vi "Digital port disable alternative functions.vi"(8 "error in (no error)":errorcluster, 10 "Lines":T1 items=["DIO1...8"=1, "DIO9...16"=2, "DIO17...24"=3, "DIO25...32"=4], 11 "Connection ID":i32) -> (0 "error out":errorcluster, 3 "connection ID out":i32)   [LabVIEW 2009, in "MicroDAQ.lvlib" / "Digital Input.lvclass"]
uses:
  <instrlib>/MicroDAQ/Channel/Digital Input/Digital Input.lvclass
  <instrlib>/MicroDAQ/Tools/Digital IO channels.ctl
  <instrlib>/MicroDAQ/Tools/DIO Alternative functions.ctl
  <instrlib>/MicroDAQ/Tools/DIO set function argument.ctl
  <instrlib>/MicroDAQ/MicroDAQ.lvlib
  <instrlib>/MicroDAQ/Mlink library wraper/mlink.lvlib
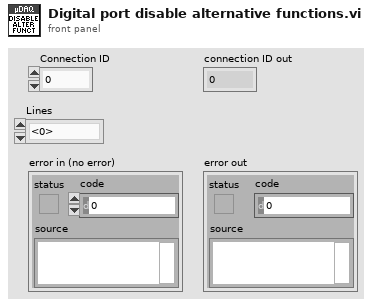
[diagram p1: front panel]
types:
  T1 = typedef "MicroDAQ.lvlib/Digital IO channels.ctl" = u8
  T2 = typedef "MicroDAQ.lvlib/DIO Alternative functions.ctl" = enum8{"None", "ENC1 (DIO1,DIO2)", "ENC2 (DIO3, DIO4)", "PWM1 (DIO10, DIO11)", "PWM2 (DIO12, DIO13)", "PWM3 (DIO14, DIO15)", "UART (DIO8-Rx, DIO9-Tx)"}
  T3 = typedef "MicroDAQ.lvlib/DIO set function argument.ctl" = enum8{"Disable", "Enable"}
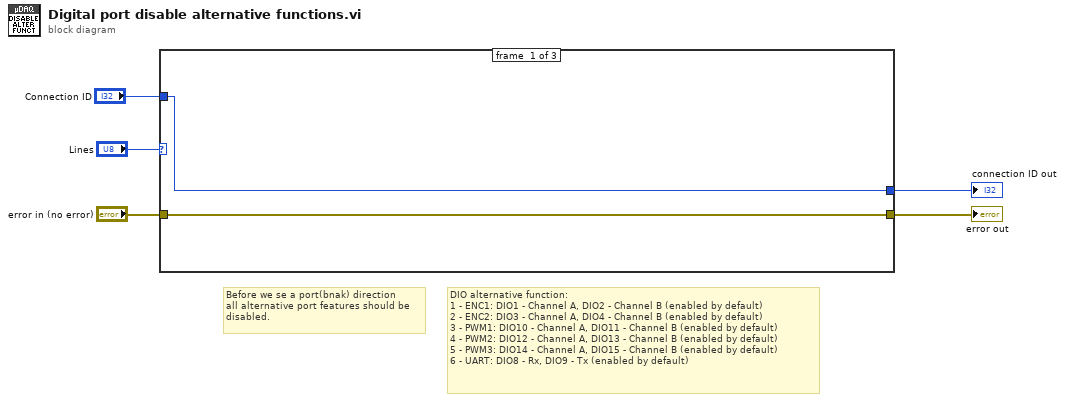
[diagram p0: block diagram]
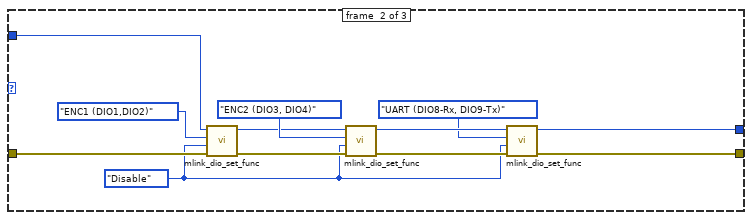
[diagram p2: hidden frame]
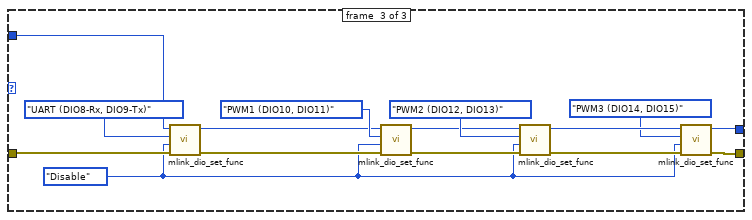
[diagram p3: hidden frame]
diagram:
  # "Before we se a port(bnak) direction\nall alternative port features should be \ndisabled."
  # "DIO alternative function:\n1 - ENC1: DIO1 - Channel A, DIO2 - Channel B (enabled by default)\n2 - ENC2: DIO3 - Channel A, DIO4 - Channel B (enabled by default)\n3 - PWM1: DIO10 - Channel A, DIO11 - Channel B (enabled by default)\n4 - PWM2: DIO12 - Channel A, DIO13 - Channel B (enabled by default)\n5 - PWM3: DIO14 - Channel A, DIO15 - Channel B (enabled by default)\n6 - UART: DIO8 - Rx, DIO9 - Tx (enabled by default)"
  n1 = case shown="2" "Lines" {
    tunnel: "Connection ID" -> [w7 w19 w23]
    tunnel: "error in (no error)" -> [w6 w18 w24]
    tunnel: [w6 w9 w26] -> w4
    tunnel: [w7 w8 w27] -> w3
    frame #0 {
    }
    frame #1 {
      w10 = DIO_set_function_argument."Disable" ("state")
      n2 = call <instrlib>:"mlink_dio_set_func.vi"("error in (no error)"=w18, "state"=w10, "function"=DIO_Alternative_functions."ENC1 (DIO1,DIO2)", "connection ID"=w19) -> ("error out"=w14:errorcluster, "connection ID out"=w15:i32)  [unwired: 6 in]
      n3 = call <instrlib>:"mlink_dio_set_func.vi"("error in (no error)"=w14, "state"=w10, "function"=DIO_Alternative_functions."ENC2 (DIO3, DIO4)", "connection ID"=w15) -> ("error out"=w12:errorcluster, "connection ID out"=w13:i32)  [unwired: 6 in]
      n4 = call <instrlib>:"mlink_dio_set_func.vi"("error in (no error)"=w12, "state"=w10, "function"=DIO_Alternative_functions."UART (DIO8-Rx, DIO9-Tx)", "connection ID"=w13) -> ("error out"=w9:errorcluster, "connection ID out"=w8:i32)  [unwired: 6 in]
    }
    frame #2 {
      w20 = DIO_set_function_argument."Disable" ("state")
      n5 = call <instrlib>:"mlink_dio_set_func.vi"("error in (no error)"=w24, "state"=w20, "function"=DIO_Alternative_functions."UART (DIO8-Rx, DIO9-Tx)", "connection ID"=w23) -> ("error out"=w25:errorcluster, "connection ID out"=w22:i32)  [unwired: 6 in]
      n6 = call <instrlib>:"mlink_dio_set_func.vi"("error in (no error)"=w25, "state"=w20, "function"=DIO_Alternative_functions."PWM1 (DIO10, DIO11)", "connection ID"=w22) -> ("error out"=w31:errorcluster, "connection ID out"=w32:i32)  [unwired: 6 in]
      n7 = call <instrlib>:"mlink_dio_set_func.vi"("error in (no error)"=w31, "state"=w20, "function"=DIO_Alternative_functions."PWM2 (DIO12, DIO13)", "connection ID"=w32) -> ("error out"=w29:errorcluster, "connection ID out"=w30:i32)  [unwired: 6 in]
      n8 = call <instrlib>:"mlink_dio_set_func.vi"("error in (no error)"=w29, "state"=w20, "function"=DIO_Alternative_functions."PWM3 (DIO14, DIO15)", "connection ID"=w30) -> ("error out"=w26:errorcluster, "connection ID out"=w27:i32)  [unwired: 6 in]
    }
  }
  "error out" <- w4
  "connection ID out" <- w3
